vi "NI VeriStand - Enable System Explorer Update Buffer Wrapper.vi"(8 "error in":errorcluster) -> (0 "error out":errorcluster)   [LabVIEW 2020, in "DSF System Explorer.lvlib"]
uses:
  DSF System Explorer.lvlib
  <vilib>/NI VeriStand/Custom Device API/Custom Device API.lvlib
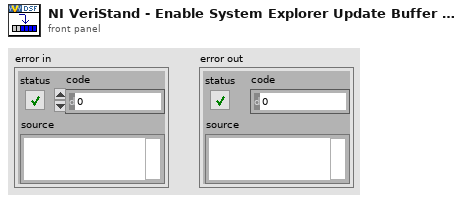
[diagram p1: front panel]
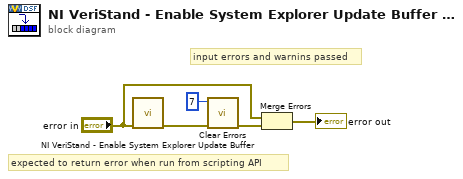
[diagram p0: block diagram]
diagram:
  # "input errors and warnins passed"
  # "expected to return error when run from scripting API"
  n1 = call <vilib>:"NI VeriStand - Enable System Explorer Update Buffer.vi"("error in (no error)"="error in") -> ("error out"=w4:errorcluster)  [unwired: 10 in]
  n2 = call <vilib>:"Clear Errors.vi"("error in (no error)"=w4, "specific error code to clear (0: all)"=7) -> ("error out"=w2:errorcluster)  [unwired: 4 in, 1 out]
  n3 = Merge Errors("error in", w2) -> (→"error out":errorcluster)
